vi "Device_Measurement_Start.vi"(2 "Device Selection":T2, 3 "Devices":T1) -> ()   [LabVIEW 2024]
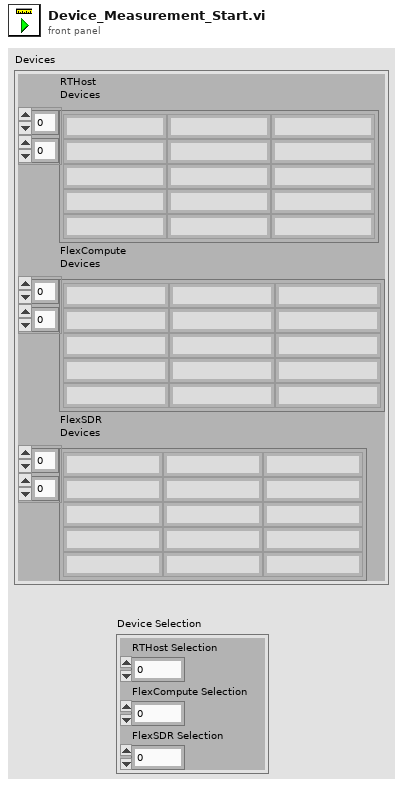
[diagram p1: front panel]
types:
  T1 = cluster{"RTHost\nDevices":string[][], "FlexCompute\nDevices":string[][], "FlexSDR\nDevices":string[][]}
  T2 = cluster{"RTHost Selection":u16, "FlexCompute Selection":u16, "FlexSDR Selection":u16}
  T3 = cluster{"SDR Config":cluster{"WRx 1\nEnable Channel":bool, "WRx 1\nIF Frequency":u16, "WRx 1\nBandwidth Mode":u16, "WRx 1\nGain Mode":u16, "WRx 1\nRSSI Threshold":dbl, "WRx 1\nGain Attenuation":i64, "WRx 2\nEnable Channel":bool, "WRx 2\nIF Frequency":u16, "WRx 2\nBandwidth Mode":u16, "WRx 2\nGain Mode":u16, "WRx 2\nRSSI Threshold":dbl, "WRx 2\nGain Attenuation":i64, "Runtime\nCalibration":bool, "Measurement\nActive":bool}, "Compute Config":cluster{"Doppler\nBypass":bool, "Trigger Type":u16, "Trigger Frequency":u16, "Pre-Trigger Time":dbl, "Post-Trigger Time":dbl}}
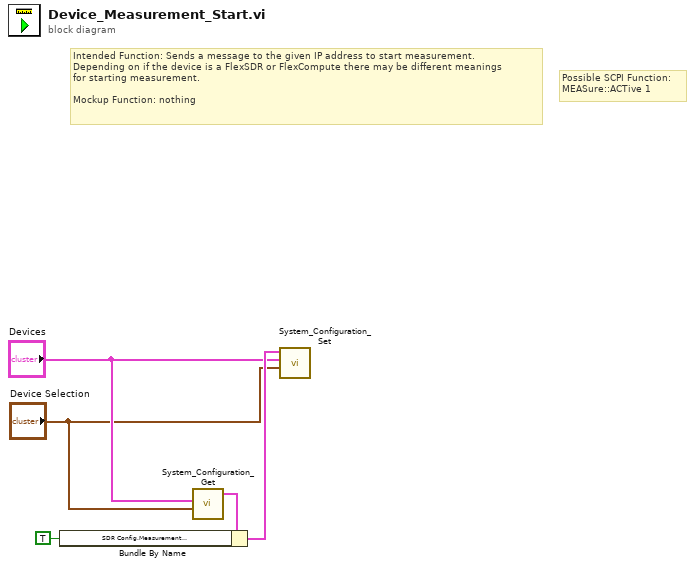
[diagram p0: block diagram]
diagram:
  # "Possible SCPI Function:\nMEASure::ACTive 1"
  # "Intended Function: Sends a message to the given IP address to start measurement.\nDepending on if the device is a FlexSDR or FlexCompute there may be different meanings\nfor starting measurement.\n\nMockup Function: nothing"
  n1 = call "System_Configuration_Get.vi"("Device Selection"="Device Selection", "Devices"="Devices") -> ("Config"=w5:T3)  [unwired: 3 in, 1 out]
  n2 = Bundle By Name(cluster=w5, "SDR Config.Measurement\nActive"=TRUE ("SDR Config.Measurement\nActive")) -> (w3:T3)
  n3 = call "System_Configuration_Set.vi"("Device Selection"="Device Selection", "Devices"="Devices", "Config"=w3) -> ()  [unwired: 4 in]
